vi "monochromatorCommandSetUnits.vi"(8 "error in":errorcluster, 10 "unit":i32(ring) items=["NM", "UM", "WN"], 11 "monochromator":refnum<k24>) -> (0 "error out":errorcluster, 3 "monochromator":refnum<k24>)   [LabVIEW 2009]
doc: "SET Wavelength UNITS"
uses:
  C:/Users/anderson.chen/Desktop/Software Development/Cornerstone Series API (LV9)/Cornerstone DLL/Cornerstone.dll
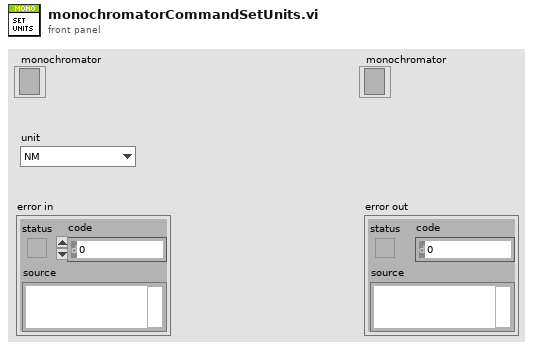
[diagram p1: front panel]
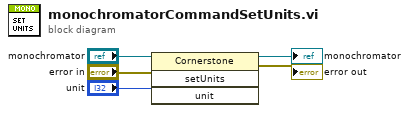
[diagram p0: block diagram]
diagram:
  n1 = invoke class="Cornerstone" method="setUnits"(reference="monochromator", error in="error in", "unit"="unit") -> (reference out=→"monochromator":refnum<k24>, error out=→"error out":errorcluster)  [unwired: 1 in, 2 out]
